vi "Write Event.vi"(7 "Event Level (Info)":T1=enum."Info", 8 "error in (no error)":errorcluster, 10 "Message":string, 11 "EventLoggingService in":refnum<class "EventLoggingService.lvclass">) -> (0 "error out":errorcluster, 3 "EventLoggingService out":refnum<class "EventLoggingService.lvclass">)   [LabVIEW 2020, in "Vecto.lvlib" / "EventLoggingService.lvclass"]
uses:
  EventLoggingService.lvclass
  Event Level.ctl
  EventLoggingService.lvclass/EventLoggingService.ctl
  EventLogHandler/EventLogHandler.lvclass
  Vecto.lvlib
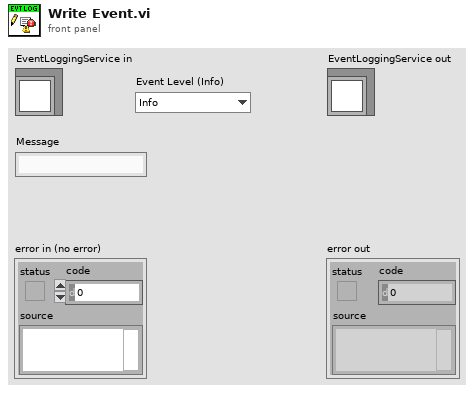
[diagram p1: front panel]
types:
  T1 = typedef "Vecto.lvlib/Event Level.ctl" = enum16{"Debug", "Info", "Warning", "Error"}
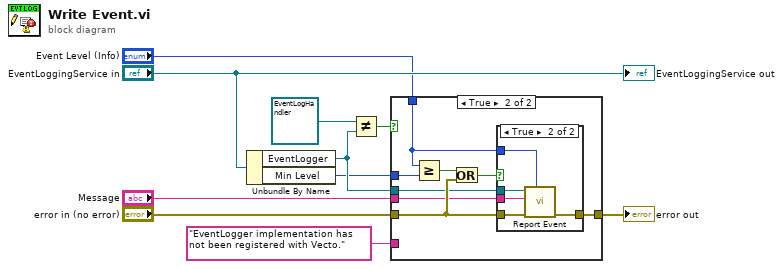
[diagram p0: block diagram]
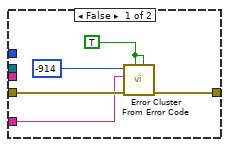
[diagram p2: hidden frame]
diagram:
  n1 = Unbundle By Name("EventLoggingService in") -> ("EventLogger"=w6:refnum<class "EventLogHandler.lvclass">, "Min Level"=w2:T1)
  n2 = Not Equal?(x=refnum<class "EventLogHandler.lvclass"> refnum, y=w6) -> (x != y?=w4:bool)
  n3 = case shown="True" w4 {
    tunnel: "Event Level (Info)" -> [_ w18]
    tunnel: "Message" -> [_ w22]
    tunnel: "error in (no error)" -> [w15 w23]
    tunnel: [w14 w21] -> w7
    tunnel: w6 -> [_ w20]
    tunnel: "EventLogger implementation has not been registered with Vecto." -> [w12 _]
    tunnel: w2 -> [_ w19]
    frame False {
      w11 = TRUE ("is warning? (False)")
      n4 = call <vilib>:"Error Cluster From Error Code.vi"("is warning? (False)"=w11, "show call chain? (False)"=w11, "error in (no error)"=w15, "error message (\"\")"=w12, "error code (0)"=-914) -> ("error out"=w14:errorcluster)  [unwired: 4 in]
    }
    frame True {
      n5 = Greater Or Equal?(x=w18, y=w19) -> (x >= y?=w17:bool)
      n6 = Or(x=w17, y=w23) -> (x .or. y?=w16:bool)
      n7 = case shown="True" w16 {
        tunnel: w22 -> [_ w29]
        tunnel: w23 -> [w24 w28]
        tunnel: [w24 w27] -> w21
        tunnel: w20 -> [_ w26]
        tunnel: w18 -> [_ w25]
        frame False {
        }
        frame True {
          n8 = call-dynamic "Report Event.vi"("Event Level (Info)"=w25, "error in (no error)"=w28, "Message"=w29, "EventLogHandler in"=w26) -> ("error out"=w27:errorcluster)  [unwired: 7 in]
        }
      }
    }
  }
  "error out" <- w7
  "EventLoggingService out" <- "EventLoggingService in"
